vi "Double to Word_ One Parameter.vi"(6 "Parameter Index":i32, 7 "Word In":u32, 8 "Param Setting":T1 {"Num Bits" min=1 max=32; "Start Bit" min=8 max=31}, 9 "NI-VS Channel":dbl) -> (1 "Word Out":u32)   [LabVIEW 2017, in "Ballard Arinc-429 Engine.lvlib"]
uses:
  RT Driver/Ballard Arinc-429 Engine.lvlib
  RT Driver/RT Controls/RT Param Setting.ctl
  Controls and Global/Start Bit.ctl
  Controls and Global/Number of Bits.ctl
  Ballard Arinc-429 Shared.lvlib
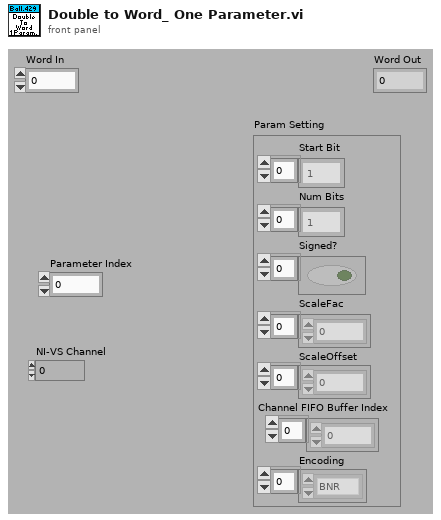
[diagram p1: front panel]
types:
  T1 = typedef "Ballard Arinc-429 Engine.lvlib/RT Param Setting.ctl" = cluster{"Start Bit":T2[], "Num Bits":T3[], "Signed?":bool[], "ScaleFac":dbl[], "ScaleOffset":dbl[], "Channel FIFO Buffer Index":i32[], "Encoding":enum16{"BNR", "BCD", "Discrete"}[]}
  T2 = typedef "Ballard Arinc-429 Shared.lvlib/Start Bit.ctl" = i32
  T3 = typedef "Ballard Arinc-429 Shared.lvlib/Number of Bits.ctl" = i32
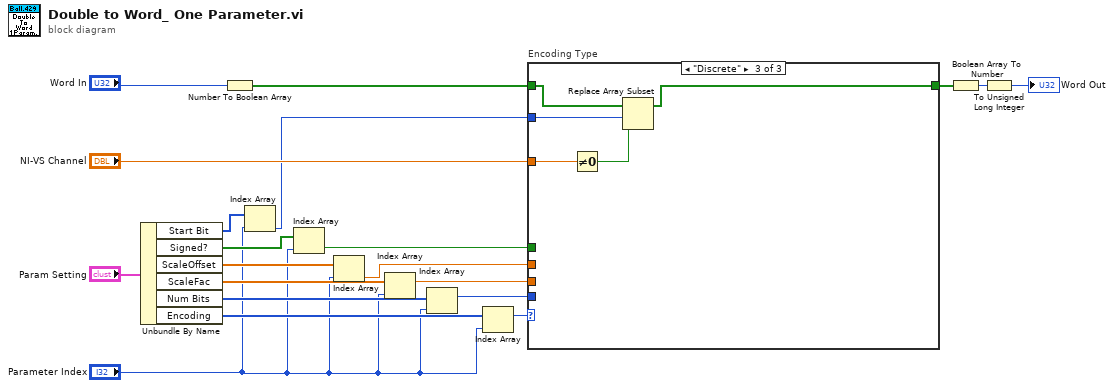
[diagram p0: block diagram]
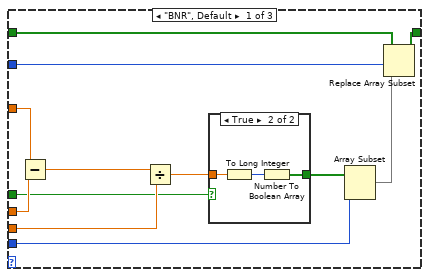
[diagram p2: hidden frame]
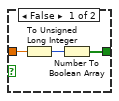
[diagram p3: hidden frame]
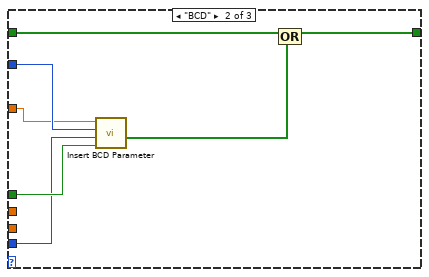
[diagram p4: hidden frame]
diagram:
  n1 = Unbundle By Name("Param Setting") -> ("Start Bit"=w15:T2[], "Signed?"=w14:bool[], "ScaleOffset"=w6:dbl[], "ScaleFac"=w19:dbl[], "Num Bits"=w20:T3[], "Encoding"=w13:enum16{"BNR", "BCD", "Discrete"}[])
  n2 = Number To Boolean Array(number="Word In") -> (Boolean array=w7:bool[])
  n3 = Index Array(array=w15, index="Parameter Index") -> (element=w10:T2)
  n4 = Index Array(array=w14, index="Parameter Index") -> (element=w9:bool)
  n5 = Index Array(array=w6, index="Parameter Index") -> (element=w5:dbl)
  n6 = Index Array(array=w19, index="Parameter Index") -> (element=w4:dbl)
  n7 = Index Array(array=w20, index="Parameter Index") -> (element=w3:T3)
  n8 = Index Array(array=w13, index="Parameter Index") -> (element=w2:enum16{"BNR", "BCD", "Discrete"})
  n9 = case "Encoding Type" shown="\"Discrete\"" w2 {
    tunnel: w4 -> [w31 _ _]
    tunnel: [w27 w44 w50] -> w18
    tunnel: w7 -> [w26 w45 w49]
    tunnel: w10 -> [w22 w41 w48]
    tunnel: w5 -> [w25 _ _]
    tunnel: w3 -> [w24 w40 _]
    tunnel: w9 -> [w23 w43 _]
    tunnel: "NI-VS Channel" -> [w21 w39 w46]
    frame "BNR", Default {
      n10 = Subtract(x=w21, y=w25) -> (x-y=w32:dbl)
      n11 = Divide(x=w32, y=w31) -> (x/y=w30:dbl)
      n12 = case shown="True" w23 {
        tunnel: w30 -> [w35 w38]
        tunnel: [w33 w36] -> w29
        frame False {
          n13 = To Unsigned Long Integer(number=w35) -> (unsigned 32bit integer=w34:u32)
          n14 = Number To Boolean Array(number=w34) -> (Boolean array=w33:bool[])
        }
        frame True {
          n15 = To Long Integer(number=w38) -> (32bit integer=w37:i32)
          n16 = Number To Boolean Array(number=w37) -> (Boolean array=w36:bool[])
        }
      }
      n17 = Array Subset(array=w29, length=w24) -> (w28:bool[])  [unwired: 1 in]
      n18 = Replace Array Subset(array=w26, new element=w28, index=w22) -> (w27:bool[])
    }
    frame "BCD" {
      n19 = call "Insert BCD Parameter.vi"("Signed?"=w43, "Number of Bits"=w40, "Start Bit"=w41, "BCD Value"=w39) -> ("BCD Mask"=w42:bool[])  [unwired: 6 in, 1 out]
      n20 = Compound Arithmetic op=OR(w45, w42) -> (w44:bool[])
    }
    frame "Discrete" {
      n21 = Not Equal To 0?(x=w46) -> (x != 0?=w47:bool)
      n22 = Replace Array Subset(array=w49, new element=w47, index=w48) -> (w50:bool[])
    }
  }
  n23 = Boolean Array To Number(Boolean array=w18) -> (number=w17:u32)
  n24 = To Unsigned Long Integer(number=w17) -> (unsigned 32bit integer=→"Word Out":u32)
